vi "Do.vi"(8 "error in (no error)":errorcluster, 10 "Actor in":refnum<class "Actor.lvclass">, 11 "Prompt User for File Path to Load From":refnum<class "Prompt User for File Path to Load From.lvclass">) -> (0 "error out":errorcluster, 2 "Actor out":refnum<class "Actor.lvclass">)   [LabVIEW 2016, in "Controller UI.lvlib" / "Prompt User for File Path to Load From.lvclass"]
uses:
  <userlib>/Common Components/Controller UI/Messages/Prompt User for Path to load/Prompt User for File Path to Load From.lvclass
  <vilib>/ActorFramework/Actor/Actor.lvclass
  <userlib>/Common Components/Controller UI/Controller UI.lvclass
  C:/Program Files (x86)/National Instruments/LabVIEW 2016/vi.lib/ActorFramework/Actor/Actor.lvclass
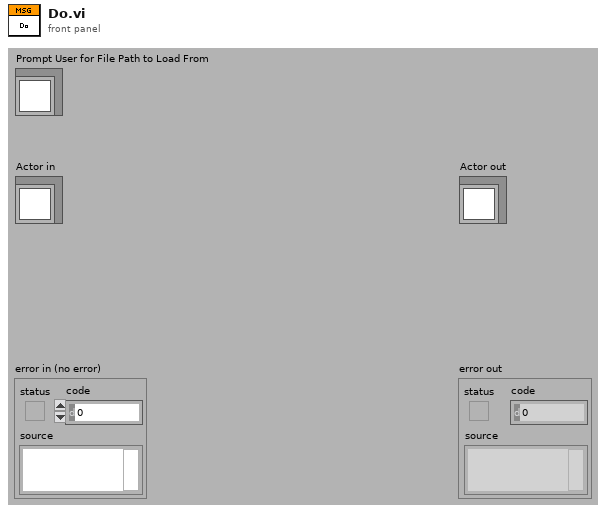
[diagram p1: front panel]
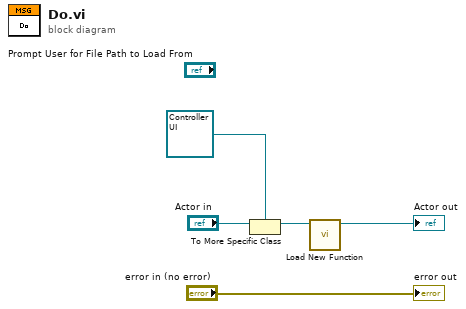
[diagram p0: block diagram]
diagram:
  n1 = To More Specific Class(target class=refnum<class "Controller UI.lvclass"> refnum ("UI.lvclass"), reference="Actor in") -> (specific class reference=w2:refnum<class "Controller UI.lvclass">)  [unwired: 1 in, 1 out]
  n2 = call-dynamic "Load New Function.vi"("UI in"=w2) -> ("UI out"=→"Actor out":refnum<class "Controller UI.lvclass">)  [unwired: 9 in, 1 out]
  "error out" <- "error in (no error)"
